vi "WriteExcel.vi"(0 "Table":string[][](table)=[["1", "2", "3", "4", "5", "6", "7", "8", "9", "10"], ["10", "11", "12", "13", "14", "15", "16", "17", "18", "19"], ["20", "21", "22", "23", "24", "25", "26", "27", "28", "29"], ["30", "31", "32", "33", "34", "35", "36", "37", "38", "39"]], 1 "是否写入":bool, 2 "数值":i8=1, 3 "路径":path) -> ()   [LabVIEW 2011]
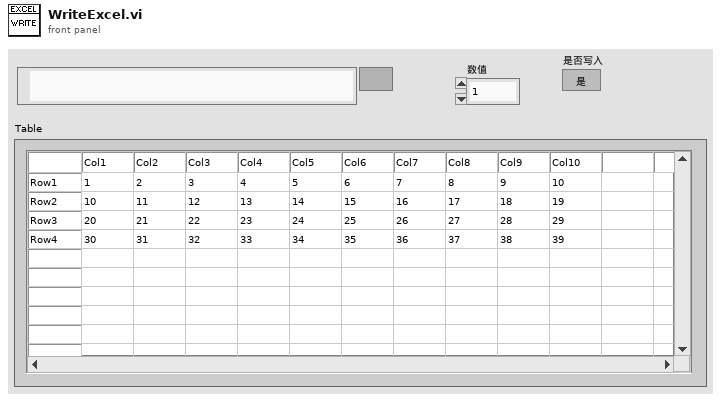
[diagram p1: front panel]
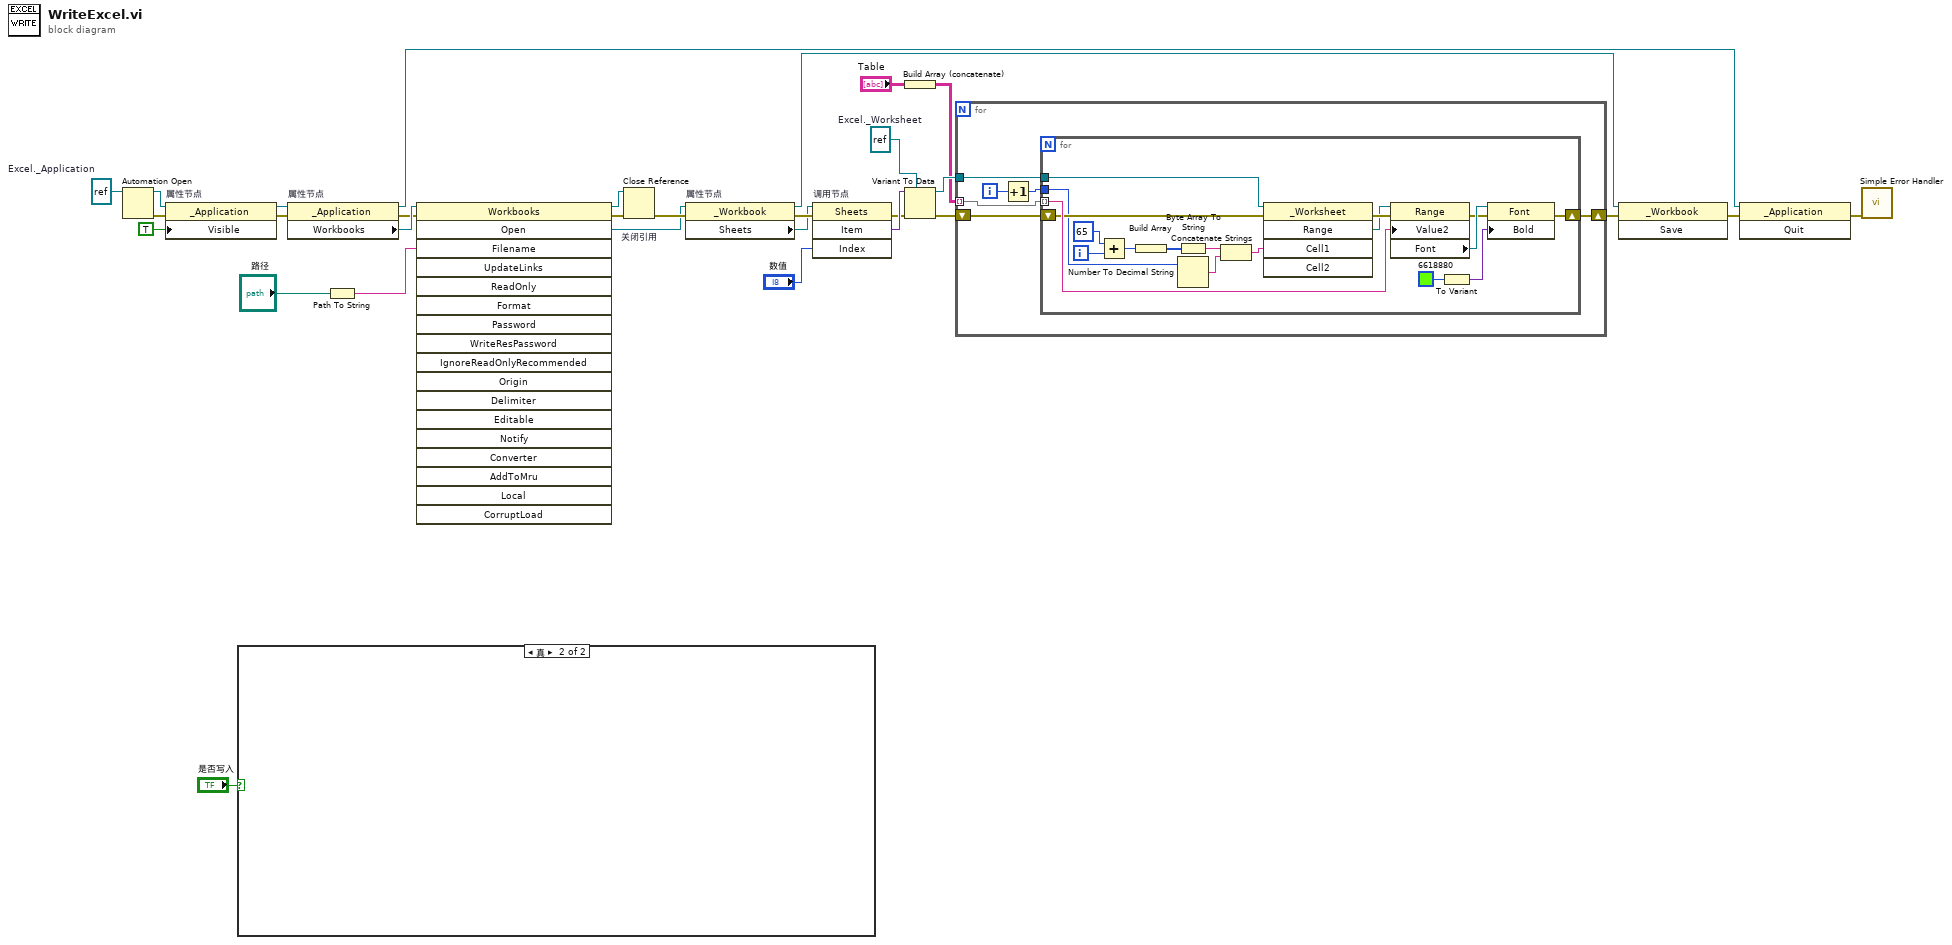
[diagram p0: block diagram]
diagram:
  w17 = refnum<k7> refnum  # Excel._Worksheet
  w28 = refnum<k7> refnum  # Excel._Application
  n1 = Automation Open(Automation Refnum=w28) -> (Automation Refnum=w29:refnum<k7>, error out=w30:errorcluster)  [unwired: 1 in, 2 out]
  n2 = property on="属性节点" class="_Application"(reference=w29, error in=w30, "Visible"=TRUE) -> (reference out=w21:refnum<k7>, error out=w23:errorcluster)
  n3 = case shown="真" "是否写入" {
    frame False {
    }
    frame True {
    }
  }
  n4 = property on="属性节点" class="_Application"(reference=w21, error in=w23) -> (reference out=w6:refnum<k7>, error out=w26:errorcluster, "Workbooks"=w27:refnum<k7>)
  n5 = Path To String(path="路径") -> (string=w10:string)
  n6 = invoke class="Workbooks" method="Open"(reference=w27, error in=w26, "Filename"=w10) -> (reference out=w24:refnum<k7>, error out=w25:errorcluster, "Open"=w19:refnum<k7>)  [unwired: 15 in, 15 out]
  n7 = Close Reference "关闭引用"(reference=w24, error in (no error)=w25) -> (error out=w20:errorcluster)
  n8 = property on="属性节点" class="_Workbook"(reference=w19, error in=w20) -> (reference out=w7:refnum<k7>, error out=w15:errorcluster, "Sheets"=w14:refnum<k7>)
  n9 = invoke on="调用节点" class="Sheets" method="Item"(reference=w14, error in=w15, "Index"="数值") -> (error out=w5:errorcluster, "Item"=w16:variant)  [unwired: 1 in, 2 out]
  n10 = Build Array (concatenate)("Table") -> (w8:string[][])
  n11 = Variant To Data(error in=w5, type=w17, Variant=w16) -> (data=w18:refnum<k7>, error out=w13:errorcluster)
  n12 = for {
    shift-right: [w35] -> w4
    shift-left: w13 -> [w36]
    tunnel: w18 -> [w34]
    tunnel: w8 -> [w31] mode=indexing
    i -> [w33]
    n13 = Increment(x=w33) -> (x+1=w32:i32)
    n14 = for {
      shift-right: [w38] -> w35
      shift-left: w36 -> [w51]
      tunnel: w34 -> [w50]
      tunnel: w32 -> [w45]
      tunnel: w31 -> [w52] mode=indexing
      i -> [w46]
      n15 = Add(x=65, y=w46) -> (x+y=w48:i32)
      n16 = Build Array(w48) -> (w47:i32[])
      n17 = Byte Array To String(unsigned byte array=w47) -> (string=w44:string)
      n18 = Number To Decimal String(number=w45) -> (decimal integer string=w43:string)  [unwired: 1 in]
      n19 = Concatenate Strings(w44, w43) -> (w42:string)
      n20 = invoke class="_Worksheet" method="Range"(reference=w50, error in=w51, "Cell1"=w42) -> (error out=w54:errorcluster, "Range"=w53:refnum<k7>)  [unwired: 2 in, 3 out]
      n21 = property class="Range"(reference=w53, error in=w54, "Value2"=w52) -> (error out=w40:errorcluster, "Font"=w41:refnum<k7>)  [unwired: 1 out]
      n22 = To Variant(anything=u32 6618880 ("颜色盒")) -> (Variant=w37:variant)
      n23 = property class="Font"(reference=w41, error in=w40, "Bold"=w37) -> (error out=w38:errorcluster)  [unwired: 1 out]
    }
  }
  n24 = invoke class="_Workbook" method="Save"(reference=w7, error in=w4) -> (error out=w3:errorcluster)  [unwired: 1 in, 2 out]
  n25 = invoke class="_Application" method="Quit"(reference=w6, error in=w3) -> (error out=w2:errorcluster)  [unwired: 1 in, 2 out]
  n26 = call <vilib>:"Simple Error Handler.vi"("error in (no error)"=w2) -> ()  [unwired: 4 in, 5 out]
